vi "Jump to Line in ATR (SubVI).vi"(8 "error in (no error)":errorcluster, 10 "Line number":i32, 11 "Table in":refnum<vi>) -> (0 "error out":errorcluster, 3 "Table out":refnum<vi>)   [LabVIEW 2017]
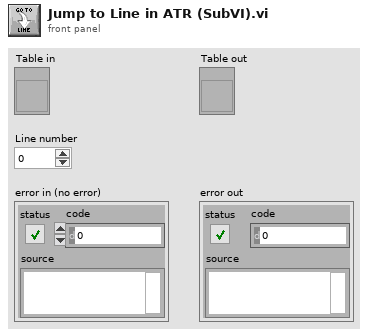
[diagram p1: front panel]
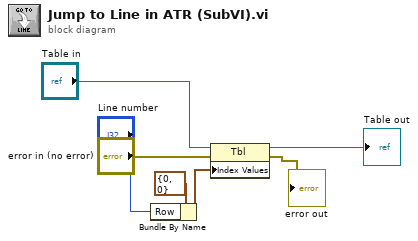
[diagram p0: block diagram]
diagram:
  n1 = Bundle By Name(cluster=cluster{"Row":i32, "Column":i32} {"Row"=0, "Column"=0} ("Edit Position"), "Row"="Line number") -> (w2:cluster{"Row":i32, "Column":i32})
  n2 = property on="Property Node" class="Tbl"(reference="Table in", error in="error in (no error)", "Index Values"=w2) -> (reference out=→"Table out":refnum<vi>, error out=→"error out":errorcluster)
